vi "ZAlign_LocalsPos.vi"(4 "rect in":T1, 5 "Max Right":u32, 6 "Grid_Size":i16, 7 "Left":u32, 9 "Height+Grid":u32, 10 "Positions+Grid+MaxRight":u32[](array[numeric]), 11 "Bottom":u32) -> (3 "rect out":T1)   [LabVIEW 2014, in "ZAlign.lvlib"]
doc: "ZAlign.lvlib:ZAlign_LocalsPos.vi\n----------------------------------------------\nLocals Rahmen berechnen.\n\nInputs:\n---------------------\n- rect in : Cluster; \n- Max Right : U32; \n- Grid_Size : I16; \n- Left : U32; \n- Height+Grid : U32; \n- Positions+Grid+MaxRight : 1DArrayOfU32; \n- Bottom : U32; \n\nOutputs:\n---------------------\n- rect out : Cluster; \n\n----------------------------------------------\n26.03.2015 jcm\nZühlke Engineering AG\nCH-8952 Schlieren\nwww.zuehlke.com"
uses:
  ZAlign.lvlib
panel:
  # "Connector Pane"
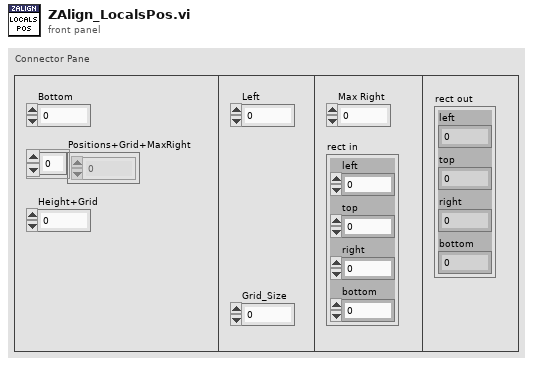
[diagram p1: front panel]
types:
  T1 = cluster{"left":i16, "top":i16, "right":i16, "bottom":i16}
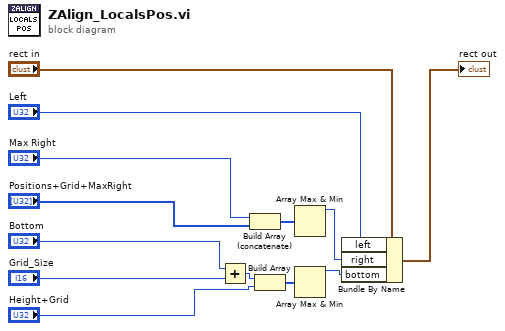
[diagram p0: block diagram]
diagram:
  n1 = Add(x="Bottom", y="Grid_Size") -> (x+y=w12:u32)
  n2 = Build Array (concatenate)("Max Right", "Positions+Grid+MaxRight") -> (w7:u32[])
  n3 = Build Array(w12, "Height+Grid") -> (w3:u32[])
  n4 = Array Max & Min(array=w7) -> (max value=w9:u32)  [unwired: 3 out]
  n5 = Array Max & Min(array=w3) -> (max value=w4:u32)  [unwired: 3 out]
  n6 = Bundle By Name(cluster="rect in", "left"="Left", "right"=w9, "bottom"=w4) -> (→"rect out":T1)
